vi "multi-function-fpga2.vi"() -> ()   [LabVIEW 2016]
uses:
  <vilib>/rvi/Emulation/niFpgaGetClockAttributes.vi
  <vilib>/rvi/Emulation/niFpgaSctlEmulationGetInTimedLoop.vi
  <vilib>/rvi/Emulation/niFpgaEmulationReportErrorSimple.vi
  <vilib>/rvi/eio/common/nirviEmuTemplateMethod_errors.vi
  <vilib>/rvi/Emulation/niFpgaCriticalErrorInLSC.vi
  <vilib>/eio/EIONode/EIONode.xnode
panel:
  out "input array":bool[](array[boolean])
  in  "Channel15":T1={"Ctrl"=enum."OFF", "high voltage"=3.5, "main input"=FALSE, "sub input"=FALSE, "low voltage"=0.0, "begin voltage"=0.0, "end voltage"=0.0, "step voltage"=0.0, "Set"=FALSE} {"step voltage" format="%#_17g"; "end voltage" format="%#_17g"; "begin voltage" format="%#_17g"; "low voltage" format="%#_17g"; "high voltage" format="%#_17g"}
  in  "Channel14":T1={"Ctrl"=enum."OFF", "high voltage"=3.5, "main input"=FALSE, "sub input"=FALSE, "low voltage"=0.0, "begin voltage"=0.0, "end voltage"=0.0, "step voltage"=0.0, "Set"=FALSE} {"step voltage" format="%#_17g"; "end voltage" format="%#_17g"; "begin voltage" format="%#_17g"; "low voltage" format="%#_17g"; "high voltage" format="%#_17g"}
  in  "Channel13":T1={"Ctrl"=enum."OFF", "high voltage"=3.5, "main input"=FALSE, "sub input"=FALSE, "low voltage"=0.0, "begin voltage"=0.0, "end voltage"=0.0, "step voltage"=0.0, "Set"=FALSE} {"step voltage" format="%#_17g"; "end voltage" format="%#_17g"; "begin voltage" format="%#_17g"; "low voltage" format="%#_17g"; "high voltage" format="%#_17g"}
  in  "Channel12":T1={"Ctrl"=enum."OFF", "high voltage"=3.5, "main input"=FALSE, "sub input"=FALSE, "low voltage"=0.0, "begin voltage"=0.0, "end voltage"=0.0, "step voltage"=0.0, "Set"=FALSE} {"step voltage" format="%#_17g"; "end voltage" format="%#_17g"; "begin voltage" format="%#_17g"; "low voltage" format="%#_17g"; "high voltage" format="%#_17g"}
  in  "Channel11":T1={"Ctrl"=enum."OFF", "high voltage"=3.5, "main input"=FALSE, "sub input"=FALSE, "low voltage"=0.0, "begin voltage"=0.0, "end voltage"=0.0, "step voltage"=0.0, "Set"=FALSE} {"step voltage" format="%#_17g"; "end voltage" format="%#_17g"; "begin voltage" format="%#_17g"; "low voltage" format="%#_17g"; "high voltage" format="%#_17g"}
  in  "Channel10":T1={"Ctrl"=enum."OFF", "high voltage"=3.5, "main input"=FALSE, "sub input"=FALSE, "low voltage"=0.0, "begin voltage"=0.0, "end voltage"=0.0, "step voltage"=0.0, "Set"=FALSE} {"step voltage" format="%#_17g"; "end voltage" format="%#_17g"; "begin voltage" format="%#_17g"; "low voltage" format="%#_17g"; "high voltage" format="%#_17g"}
  in  "Channel9":T1={"Ctrl"=enum."OFF", "high voltage"=3.5, "main input"=FALSE, "sub input"=FALSE, "low voltage"=0.0, "begin voltage"=0.0, "end voltage"=0.0, "step voltage"=0.0, "Set"=FALSE} {"step voltage" format="%#_17g"; "end voltage" format="%#_17g"; "begin voltage" format="%#_17g"; "low voltage" format="%#_17g"; "high voltage" format="%#_17g"}
  in  "Channel8":T1={"Ctrl"=enum."OFF", "high voltage"=3.5, "main input"=FALSE, "sub input"=FALSE, "low voltage"=0.0, "begin voltage"=0.0, "end voltage"=0.0, "step voltage"=0.0, "Set"=FALSE} {"step voltage" format="%#_17g"; "end voltage" format="%#_17g"; "begin voltage" format="%#_17g"; "low voltage" format="%#_17g"; "high voltage" format="%#_17g"}
  in  "Channel7":T1={"Ctrl"=enum."OFF", "high voltage"=3.5, "main input"=FALSE, "sub input"=FALSE, "low voltage"=0.0, "begin voltage"=0.0, "end voltage"=0.0, "step voltage"=0.0, "Set"=FALSE} {"step voltage" format="%#_17g"; "end voltage" format="%#_17g"; "begin voltage" format="%#_17g"; "low voltage" format="%#_17g"; "high voltage" format="%#_17g"}
  in  "Channel6":T1={"Ctrl"=enum."OFF", "high voltage"=3.5, "main input"=FALSE, "sub input"=FALSE, "low voltage"=0.0, "begin voltage"=0.0, "end voltage"=0.0, "step voltage"=0.0, "Set"=FALSE} {"step voltage" format="%#_17g"; "end voltage" format="%#_17g"; "begin voltage" format="%#_17g"; "low voltage" format="%#_17g"; "high voltage" format="%#_17g"}
  in  "Channel5":T1={"Ctrl"=enum."OFF", "high voltage"=3.5, "main input"=FALSE, "sub input"=FALSE, "low voltage"=0.0, "begin voltage"=0.0, "end voltage"=0.0, "step voltage"=0.0, "Set"=FALSE} {"step voltage" format="%#_17g"; "end voltage" format="%#_17g"; "begin voltage" format="%#_17g"; "low voltage" format="%#_17g"; "high voltage" format="%#_17g"}
  in  "Channel4":T1={"Ctrl"=enum."OFF", "high voltage"=3.5, "main input"=FALSE, "sub input"=FALSE, "low voltage"=0.0, "begin voltage"=0.0, "end voltage"=0.0, "step voltage"=0.0, "Set"=FALSE} {"step voltage" format="%#_17g"; "end voltage" format="%#_17g"; "begin voltage" format="%#_17g"; "low voltage" format="%#_17g"; "high voltage" format="%#_17g"}
  in  "Channel3":T1={"Ctrl"=enum."OFF", "high voltage"=3.5, "main input"=FALSE, "sub input"=FALSE, "low voltage"=0.0, "begin voltage"=0.0, "end voltage"=0.0, "step voltage"=0.0, "Set"=FALSE} {"step voltage" format="%#_17g"; "end voltage" format="%#_17g"; "begin voltage" format="%#_17g"; "low voltage" format="%#_17g"; "high voltage" format="%#_17g"}
  in  "Channel2":T1={"Ctrl"=enum."OFF", "high voltage"=3.5, "main input"=FALSE, "sub input"=FALSE, "low voltage"=0.0, "begin voltage"=0.0, "end voltage"=0.0, "step voltage"=0.0, "Set"=FALSE} {"step voltage" format="%#_17g"; "end voltage" format="%#_17g"; "begin voltage" format="%#_17g"; "low voltage" format="%#_17g"; "high voltage" format="%#_17g"}
  in  "Channel1":T1={"Ctrl"=enum."OFF", "high voltage"=3.5, "main input"=FALSE, "sub input"=FALSE, "low voltage"=0.0, "begin voltage"=0.0, "end voltage"=0.0, "step voltage"=0.0, "Set"=FALSE} {"step voltage" format="%#_17g"; "end voltage" format="%#_17g"; "begin voltage" format="%#_17g"; "low voltage" format="%#_17g"; "high voltage" format="%#_17g"}
  in  "Channel0":T1={"Ctrl"=enum."OFF", "high voltage"=3.5, "main input"=FALSE, "sub input"=FALSE, "low voltage"=0.0, "begin voltage"=0.0, "end voltage"=0.0, "step voltage"=0.0, "Set"=FALSE} {"step voltage" format="%#_17g"; "end voltage" format="%#_17g"; "begin voltage" format="%#_17g"; "low voltage" format="%#_17g"; "high voltage" format="%#_17g"}
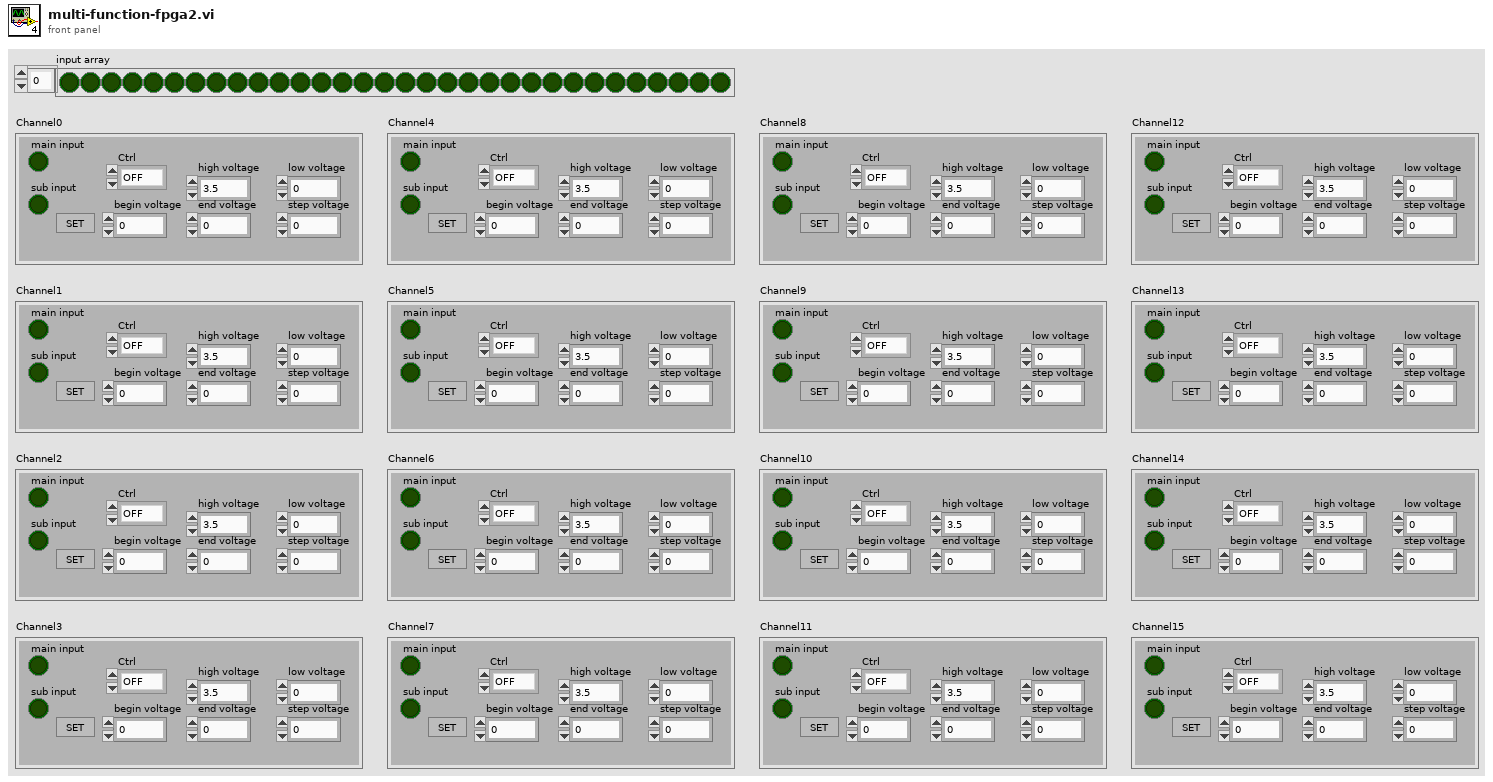
[diagram p1: front panel]
types:
  T1 = cluster{"Ctrl":enum16{"OFF", "SWITCH", "AND GATE", "OR GATE", "ITERATION"}, "high voltage":sgl, "main input":bool, "sub input":bool, "low voltage":sgl, "begin voltage":sgl, "end voltage":sgl, "step voltage":sgl, "Set":bool}
  T2 = enum16{"OFF", "SWITCH", "AND GATE", "OR GATE", "ITERATION"}
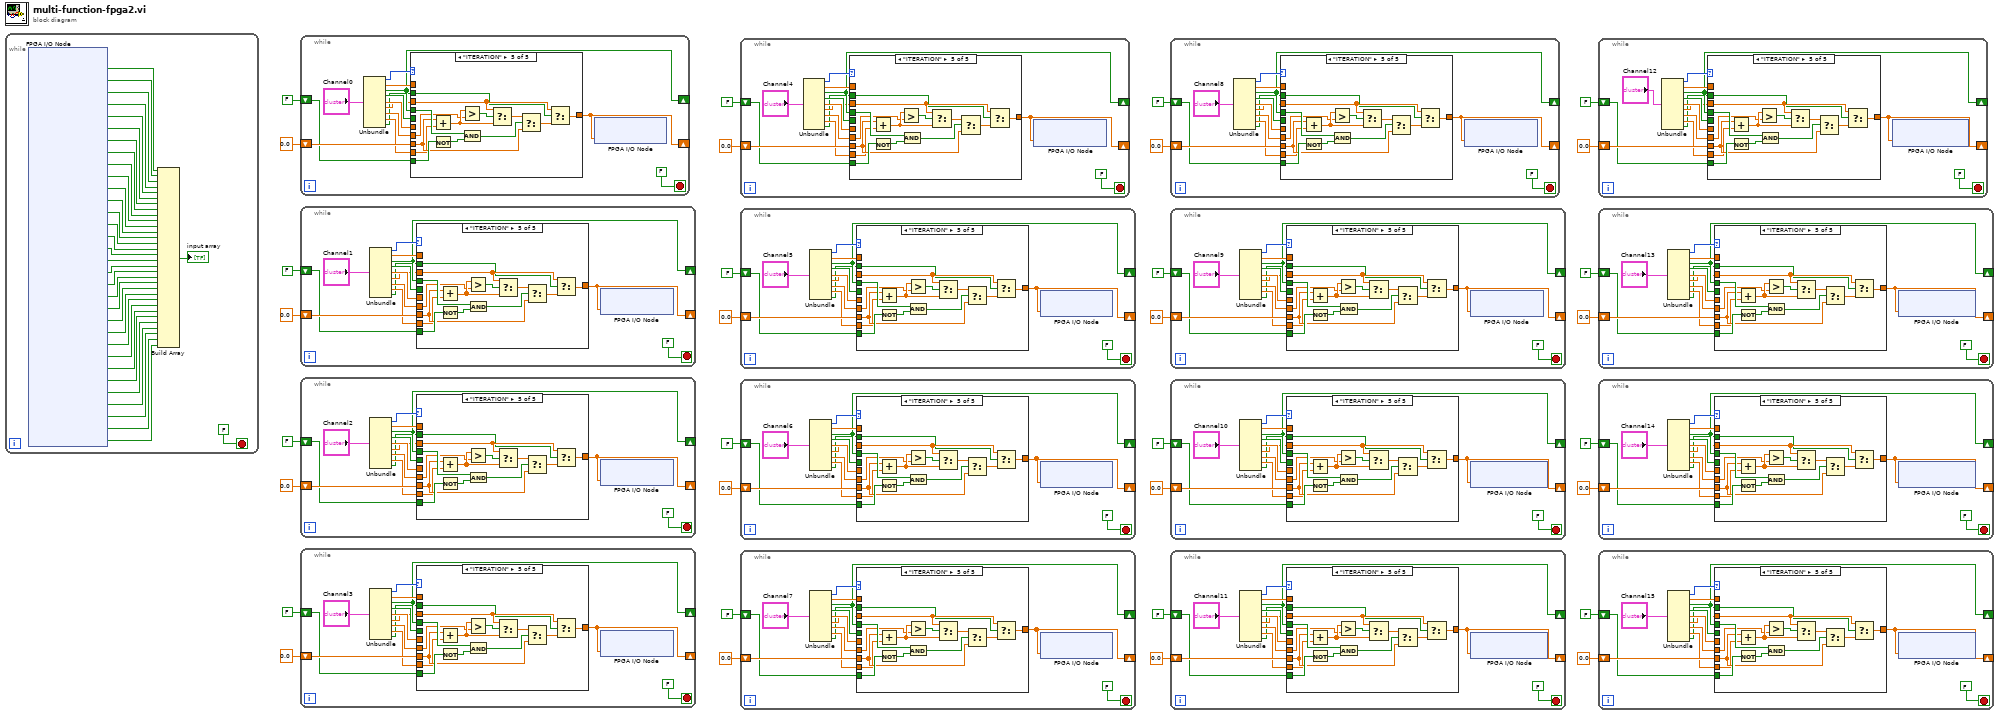
[diagram p0: block diagram]
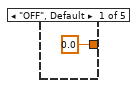
[diagram p2: hidden frame]
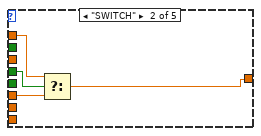
[diagram p3: hidden frame]
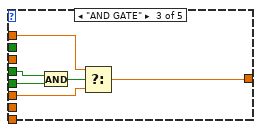
[diagram p4: hidden frame]
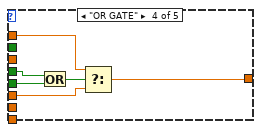
[diagram p5: hidden frame]
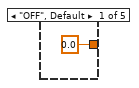
[diagram p6: hidden frame]
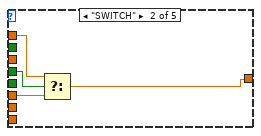
[diagram p7: hidden frame]
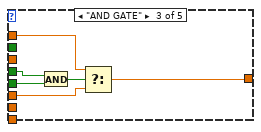
[diagram p8: hidden frame]
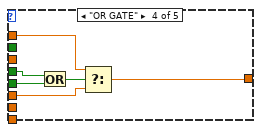
[diagram p9: hidden frame]
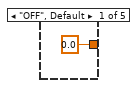
[diagram p10: hidden frame]
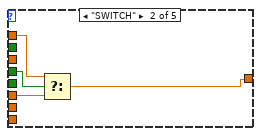
[diagram p11: hidden frame]
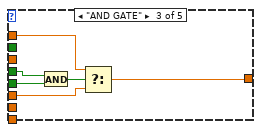
[diagram p12: hidden frame]
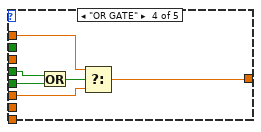
[diagram p13: hidden frame]
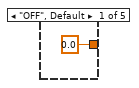
[diagram p14: hidden frame]
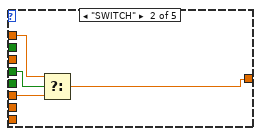
[diagram p15: hidden frame]
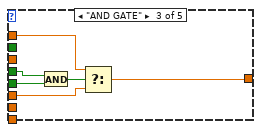
[diagram p16: hidden frame]
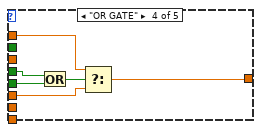
[diagram p17: hidden frame]
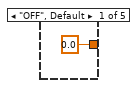
[diagram p18: hidden frame]
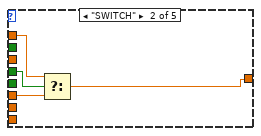
[diagram p19: hidden frame]
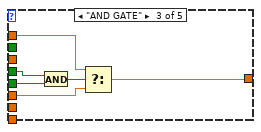
[diagram p20: hidden frame]
diagram:
  n1 = while {
    stop <- FALSE stop-if-true
    n2 = xnode "FPGA I/O Node"() -> ("Mod2/DIO0"=w65:bool, "Mod2/DIO1"=w64:bool, "Mod2/DIO2"=w63:bool, "Mod2/DIO3"=w62:bool, "Mod2/DIO4"=w61:bool, "Mod2/DIO5"=w60:bool, "Mod2/DIO6"=w59:bool, "Mod2/DIO7"=w58:bool, "Mod2/DIO8"=w57:bool, "Mod2/DIO9"=w56:bool, "Mod2/DIO10"=w55:bool, "Mod2/DIO11"=w54:bool, "Mod2/DIO12"=w53:bool, "Mod2/DIO13"=w52:bool, "Mod2/DIO14"=w51:bool, "Mod2/DIO15"=w50:bool, "Mod2/DIO16"=w49:bool, "Mod2/DIO17"=w48:bool, "Mod2/DIO18"=w47:bool, "Mod2/DIO19"=w46:bool, "Mod2/DIO20"=w45:bool, "Mod2/DIO21"=w44:bool, "Mod2/DIO22"=w43:bool, "Mod2/DIO23"=w42:bool, "Mod2/DIO24"=w41:bool, "Mod2/DIO25"=w40:bool, "Mod2/DIO26"=w39:bool, "Mod2/DIO27"=w38:bool, "Mod2/DIO28"=w37:bool, "Mod2/DIO29"=w36:bool, "Mod2/DIO30"=w35:bool, "Mod2/DIO31"=w34:bool)  [unwired: 32 in, 32 out]
    n3 = Build Array(w65, w64, w63, w62, w61, w60, w59, w58, w57, w56, w55, w54, w53, w52, w51, w50, w49, w48, w47, w46, w45, w44, w43, w42, w41, w40, w39, w38, w37, w36, w35, w34) -> (→"input array":bool[])
  }
  n4 = while {
    shift-right: [w78] -> _
    shift-left: sgl 0.0 -> [w79]
    shift-right: [w72] -> _
    shift-left: FALSE -> [w77]
    stop <- FALSE stop-if-true
    n5 = Unbundle("Channel0") -> ("Ctrl"=w75:T2, "high voltage"=w74:sgl, "main input"=w72:bool, "sub input"=w71:bool, "low voltage"=w73:sgl, "begin voltage"=w68:sgl, "end voltage"=w69:sgl, "step voltage"=w70:sgl, "Set"=w67:bool)
    n6 = case shown="\"ITERATION\"" w75 {
      tunnel: w71 -> [_ _ w90 w96 _]
      tunnel: w72 -> [_ w84 w91 w97 w110]
      tunnel: [sgl 0.0 ("Mod4/AO0") w85 w88 w94 w102] -> w78
      tunnel: w74 -> [_ w83 w87 w93 _]
      tunnel: w73 -> [_ w82 w86 w92 _]
      tunnel: w79 -> [_ _ _ _ w104]
      tunnel: w77 -> [_ _ _ _ w111]
      tunnel: w70 -> [_ _ _ _ w101]
      tunnel: w69 -> [_ _ _ _ w100]
      tunnel: w68 -> [_ _ _ _ w99]
      tunnel: w67 -> [_ _ _ _ w98]
      frame "OFF", Default {
      }
      frame "SWITCH" {
        n7 = Select(t=w83, s=w84, f=w82) -> (s? t:f=w85:sgl)
      }
      frame "AND GATE" {
        n8 = And(x=w91, y=w90) -> (x .and. y?=w89:bool)
        n9 = Select(t=w87, s=w89, f=w86) -> (s? t:f=w88:sgl)
      }
      frame "OR GATE" {
        n10 = Or(x=w97, y=w96) -> (x .or. y?=w95:bool)
        n11 = Select(t=w93, s=w95, f=w92) -> (s? t:f=w94:sgl)
      }
      frame "ITERATION" {
        n12 = Add(x=w104, y=w101) -> (x+y=w106:sgl)
        n13 = Not(x=w111) -> (.not. x?=w109:bool)
        n14 = Greater?(x=w106, y=w100) -> (0:w107:bool)
        n15 = And(x=w110, y=w109) -> (x .and. y?=w108:bool)
        n16 = Select(t=w99, s=w107, f=w106) -> (s? t:f=w105:sgl)
        n17 = Select(t=w105, s=w108, f=w104) -> (s? t:f=w103:sgl)
        n18 = Select(t=w99, s=w98, f=w103) -> (s? t:f=w102:sgl)
      }
    }
    n19 = xnode "FPGA I/O Node"("Mod4/AO0"=w78) -> ()  [unwired: 1 in, 1 out]
  }
  n20 = while {
    shift-right: [w123] -> _
    shift-left: sgl 0.0 -> [w124]
    shift-right: [w117] -> _
    shift-left: FALSE -> [w122]
    stop <- FALSE stop-if-true
    n21 = Unbundle("Channel1") -> ("Ctrl"=w120:T2, "high voltage"=w119:sgl, "main input"=w117:bool, "sub input"=w116:bool, "low voltage"=w118:sgl, "begin voltage"=w113:sgl, "end voltage"=w114:sgl, "step voltage"=w115:sgl, "Set"=w112:bool)
    n22 = case shown="\"ITERATION\"" w120 {
      tunnel: w116 -> [_ _ w135 w141 _]
      tunnel: w117 -> [_ w129 w136 w142 w155]
      tunnel: [sgl 0.0 ("Mod4/AO0") w130 w133 w139 w147] -> w123
      tunnel: w119 -> [_ w128 w132 w138 _]
      tunnel: w118 -> [_ w127 w131 w137 _]
      tunnel: w124 -> [_ _ _ _ w149]
      tunnel: w122 -> [_ _ _ _ w156]
      tunnel: w115 -> [_ _ _ _ w146]
      tunnel: w114 -> [_ _ _ _ w145]
      tunnel: w113 -> [_ _ _ _ w144]
      tunnel: w112 -> [_ _ _ _ w143]
      frame "OFF", Default {
      }
      frame "SWITCH" {
        n23 = Select(t=w128, s=w129, f=w127) -> (s? t:f=w130:sgl)
      }
      frame "AND GATE" {
        n24 = And(x=w136, y=w135) -> (x .and. y?=w134:bool)
        n25 = Select(t=w132, s=w134, f=w131) -> (s? t:f=w133:sgl)
      }
      frame "OR GATE" {
        n26 = Or(x=w142, y=w141) -> (x .or. y?=w140:bool)
        n27 = Select(t=w138, s=w140, f=w137) -> (s? t:f=w139:sgl)
      }
      frame "ITERATION" {
        n28 = Add(x=w149, y=w146) -> (x+y=w151:sgl)
        n29 = Not(x=w156) -> (.not. x?=w154:bool)
        n30 = Greater?(x=w151, y=w145) -> (0:w152:bool)
        n31 = And(x=w155, y=w154) -> (x .and. y?=w153:bool)
        n32 = Select(t=w144, s=w152, f=w151) -> (s? t:f=w150:sgl)
        n33 = Select(t=w150, s=w153, f=w149) -> (s? t:f=w148:sgl)
        n34 = Select(t=w144, s=w143, f=w148) -> (s? t:f=w147:sgl)
      }
    }
    n35 = xnode "FPGA I/O Node"("Mod4/AO1"=w123) -> ()  [unwired: 1 in, 1 out]
  }
  n36 = while {
    shift-right: [w168] -> _
    shift-left: sgl 0.0 -> [w169]
    shift-right: [w162] -> _
    shift-left: FALSE -> [w167]
    stop <- FALSE stop-if-true
    n37 = Unbundle("Channel2") -> ("Ctrl"=w165:T2, "high voltage"=w164:sgl, "main input"=w162:bool, "sub input"=w161:bool, "low voltage"=w163:sgl, "begin voltage"=w158:sgl, "end voltage"=w159:sgl, "step voltage"=w160:sgl, "Set"=w157:bool)
    n38 = case shown="\"ITERATION\"" w165 {
      tunnel: w161 -> [_ _ w180 w186 _]
      tunnel: w162 -> [_ w174 w181 w187 w200]
      tunnel: [sgl 0.0 ("Mod4/AO0") w175 w178 w184 w192] -> w168
      tunnel: w164 -> [_ w173 w177 w183 _]
      tunnel: w163 -> [_ w172 w176 w182 _]
      tunnel: w169 -> [_ _ _ _ w194]
      tunnel: w167 -> [_ _ _ _ w201]
      tunnel: w160 -> [_ _ _ _ w191]
      tunnel: w159 -> [_ _ _ _ w190]
      tunnel: w158 -> [_ _ _ _ w189]
      tunnel: w157 -> [_ _ _ _ w188]
      frame "OFF", Default {
      }
      frame "SWITCH" {
        n39 = Select(t=w173, s=w174, f=w172) -> (s? t:f=w175:sgl)
      }
      frame "AND GATE" {
        n40 = And(x=w181, y=w180) -> (x .and. y?=w179:bool)
        n41 = Select(t=w177, s=w179, f=w176) -> (s? t:f=w178:sgl)
      }
      frame "OR GATE" {
        n42 = Or(x=w187, y=w186) -> (x .or. y?=w185:bool)
        n43 = Select(t=w183, s=w185, f=w182) -> (s? t:f=w184:sgl)
      }
      frame "ITERATION" {
        n44 = Add(x=w194, y=w191) -> (x+y=w196:sgl)
        n45 = Not(x=w201) -> (.not. x?=w199:bool)
        n46 = Greater?(x=w196, y=w190) -> (0:w197:bool)
        n47 = And(x=w200, y=w199) -> (x .and. y?=w198:bool)
        n48 = Select(t=w189, s=w197, f=w196) -> (s? t:f=w195:sgl)
        n49 = Select(t=w195, s=w198, f=w194) -> (s? t:f=w193:sgl)
        n50 = Select(t=w189, s=w188, f=w193) -> (s? t:f=w192:sgl)
      }
    }
    n51 = xnode "FPGA I/O Node"("Mod4/AO2"=w168) -> ()  [unwired: 1 in, 1 out]
  }
  n52 = while {
    shift-right: [w213] -> _
    shift-left: sgl 0.0 -> [w214]
    shift-right: [w207] -> _
    shift-left: FALSE -> [w212]
    stop <- FALSE stop-if-true
    n53 = Unbundle("Channel3") -> ("Ctrl"=w210:T2, "high voltage"=w209:sgl, "main input"=w207:bool, "sub input"=w206:bool, "low voltage"=w208:sgl, "begin voltage"=w203:sgl, "end voltage"=w204:sgl, "step voltage"=w205:sgl, "Set"=w202:bool)
    n54 = case shown="\"ITERATION\"" w210 {
      tunnel: w206 -> [_ _ w225 w231 _]
      tunnel: w207 -> [_ w219 w226 w232 w245]
      tunnel: [sgl 0.0 ("Mod4/AO0") w220 w223 w229 w237] -> w213
      tunnel: w209 -> [_ w218 w222 w228 _]
      tunnel: w208 -> [_ w217 w221 w227 _]
      tunnel: w214 -> [_ _ _ _ w239]
      tunnel: w212 -> [_ _ _ _ w246]
      tunnel: w205 -> [_ _ _ _ w236]
      tunnel: w204 -> [_ _ _ _ w235]
      tunnel: w203 -> [_ _ _ _ w234]
      tunnel: w202 -> [_ _ _ _ w233]
      frame "OFF", Default {
      }
      frame "SWITCH" {
        n55 = Select(t=w218, s=w219, f=w217) -> (s? t:f=w220:sgl)
      }
      frame "AND GATE" {
        n56 = And(x=w226, y=w225) -> (x .and. y?=w224:bool)
        n57 = Select(t=w222, s=w224, f=w221) -> (s? t:f=w223:sgl)
      }
      frame "OR GATE" {
        n58 = Or(x=w232, y=w231) -> (x .or. y?=w230:bool)
        n59 = Select(t=w228, s=w230, f=w227) -> (s? t:f=w229:sgl)
      }
      frame "ITERATION" {
        n60 = Add(x=w239, y=w236) -> (x+y=w241:sgl)
        n61 = Not(x=w246) -> (.not. x?=w244:bool)
        n62 = Greater?(x=w241, y=w235) -> (0:w242:bool)
        n63 = And(x=w245, y=w244) -> (x .and. y?=w243:bool)
        n64 = Select(t=w234, s=w242, f=w241) -> (s? t:f=w240:sgl)
        n65 = Select(t=w240, s=w243, f=w239) -> (s? t:f=w238:sgl)
        n66 = Select(t=w234, s=w233, f=w238) -> (s? t:f=w237:sgl)
      }
    }
    n67 = xnode "FPGA I/O Node"("Mod4/AO3"=w213) -> ()  [unwired: 1 in, 1 out]
  }
  n68 = while {
    shift-right: [w258] -> _
    shift-left: sgl 0.0 -> [w259]
    shift-right: [w252] -> _
    shift-left: FALSE -> [w257]
    stop <- FALSE stop-if-true
    n69 = Unbundle("Channel4") -> ("Ctrl"=w255:T2, "high voltage"=w254:sgl, "main input"=w252:bool, "sub input"=w251:bool, "low voltage"=w253:sgl, "begin voltage"=w248:sgl, "end voltage"=w249:sgl, "step voltage"=w250:sgl, "Set"=w247:bool)
    n70 = case shown="\"ITERATION\"" w255 {
      tunnel: w251 -> [_ _ w270 w276 _]
      tunnel: w252 -> [_ w264 w271 w277 w290]
      tunnel: [sgl 0.0 ("Mod4/AO0") w265 w268 w274 w282] -> w258
      tunnel: w254 -> [_ w263 w267 w273 _]
      tunnel: w253 -> [_ w262 w266 w272 _]
      tunnel: w259 -> [_ _ _ _ w284]
      tunnel: w257 -> [_ _ _ _ w291]
      tunnel: w250 -> [_ _ _ _ w281]
      tunnel: w249 -> [_ _ _ _ w280]
      tunnel: w248 -> [_ _ _ _ w279]
      tunnel: w247 -> [_ _ _ _ w278]
      frame "OFF", Default {
      }
      frame "SWITCH" {
        n71 = Select(t=w263, s=w264, f=w262) -> (s? t:f=w265:sgl)
      }
      frame "AND GATE" {
        n72 = And(x=w271, y=w270) -> (x .and. y?=w269:bool)
        n73 = Select(t=w267, s=w269, f=w266) -> (s? t:f=w268:sgl)
      }
      frame "OR GATE" {
        n74 = Or(x=w277, y=w276) -> (x .or. y?=w275:bool)
        n75 = Select(t=w273, s=w275, f=w272) -> (s? t:f=w274:sgl)
      }
      frame "ITERATION" {
        n76 = Add(x=w284, y=w281) -> (x+y=w286:sgl)
        n77 = Not(x=w291) -> (.not. x?=w289:bool)
        n78 = Greater?(x=w286, y=w280) -> (0:w287:bool)
        n79 = And(x=w290, y=w289) -> (x .and. y?=w288:bool)
        n80 = Select(t=w279, s=w287, f=w286) -> (s? t:f=w285:sgl)
        n81 = Select(t=w285, s=w288, f=w284) -> (s? t:f=w283:sgl)
        n82 = Select(t=w279, s=w278, f=w283) -> (s? t:f=w282:sgl)
      }
    }
    n83 = xnode "FPGA I/O Node"("Mod4/AO4"=w258) -> ()  [unwired: 1 in, 1 out]
  }
  n84 = while {
    shift-right: [w303] -> _
    shift-left: sgl 0.0 -> [w304]
    shift-right: [w297] -> _
    shift-left: FALSE -> [w302]
    stop <- FALSE stop-if-true
    n85 = Unbundle("Channel5") -> ("Ctrl"=w300:T2, "high voltage"=w299:sgl, "main input"=w297:bool, "sub input"=w296:bool, "low voltage"=w298:sgl, "begin voltage"=w293:sgl, "end voltage"=w294:sgl, "step voltage"=w295:sgl, "Set"=w292:bool)
    n86 = case shown="\"ITERATION\"" w300 {
      tunnel: w296 -> [_ _ w315 w321 _]
      tunnel: w297 -> [_ w309 w316 w322 w335]
      tunnel: [sgl 0.0 ("Mod4/AO0") w310 w313 w319 w327] -> w303
      tunnel: w299 -> [_ w308 w312 w318 _]
      tunnel: w298 -> [_ w307 w311 w317 _]
      tunnel: w304 -> [_ _ _ _ w329]
      tunnel: w302 -> [_ _ _ _ w336]
      tunnel: w295 -> [_ _ _ _ w326]
      tunnel: w294 -> [_ _ _ _ w325]
      tunnel: w293 -> [_ _ _ _ w324]
      tunnel: w292 -> [_ _ _ _ w323]
      frame "OFF", Default {
      }
      frame "SWITCH" {
        n87 = Select(t=w308, s=w309, f=w307) -> (s? t:f=w310:sgl)
      }
      frame "AND GATE" {
        n88 = And(x=w316, y=w315) -> (x .and. y?=w314:bool)
        n89 = Select(t=w312, s=w314, f=w311) -> (s? t:f=w313:sgl)
      }
      frame "OR GATE" {
        n90 = Or(x=w322, y=w321) -> (x .or. y?=w320:bool)
        n91 = Select(t=w318, s=w320, f=w317) -> (s? t:f=w319:sgl)
      }
      frame "ITERATION" {
        n92 = Add(x=w329, y=w326) -> (x+y=w331:sgl)
        n93 = Not(x=w336) -> (.not. x?=w334:bool)
        n94 = Greater?(x=w331, y=w325) -> (0:w332:bool)
        n95 = And(x=w335, y=w334) -> (x .and. y?=w333:bool)
        n96 = Select(t=w324, s=w332, f=w331) -> (s? t:f=w330:sgl)
        n97 = Select(t=w330, s=w333, f=w329) -> (s? t:f=w328:sgl)
        n98 = Select(t=w324, s=w323, f=w328) -> (s? t:f=w327:sgl)
      }
    }
    n99 = xnode "FPGA I/O Node"("Mod4/AO5"=w303) -> ()  [unwired: 1 in, 1 out]
  }
  n100 = while {
    shift-right: [w348] -> _
    shift-left: sgl 0.0 -> [w349]
    shift-right: [w342] -> _
    shift-left: FALSE -> [w347]
    stop <- FALSE stop-if-true
    n101 = Unbundle("Channel6") -> ("Ctrl"=w345:T2, "high voltage"=w344:sgl, "main input"=w342:bool, "sub input"=w341:bool, "low voltage"=w343:sgl, "begin voltage"=w338:sgl, "end voltage"=w339:sgl, "step voltage"=w340:sgl, "Set"=w337:bool)
    n102 = case shown="\"ITERATION\"" w345 {
      tunnel: w341 -> [_ _ w360 w366 _]
      tunnel: w342 -> [_ w354 w361 w367 w380]
      tunnel: [sgl 0.0 ("Mod4/AO0") w355 w358 w364 w372] -> w348
      tunnel: w344 -> [_ w353 w357 w363 _]
      tunnel: w343 -> [_ w352 w356 w362 _]
      tunnel: w349 -> [_ _ _ _ w374]
      tunnel: w347 -> [_ _ _ _ w381]
      tunnel: w340 -> [_ _ _ _ w371]
      tunnel: w339 -> [_ _ _ _ w370]
      tunnel: w338 -> [_ _ _ _ w369]
      tunnel: w337 -> [_ _ _ _ w368]
      frame "OFF", Default {
      }
      frame "SWITCH" {
        n103 = Select(t=w353, s=w354, f=w352) -> (s? t:f=w355:sgl)
      }
      frame "AND GATE" {
        n104 = And(x=w361, y=w360) -> (x .and. y?=w359:bool)
        n105 = Select(t=w357, s=w359, f=w356) -> (s? t:f=w358:sgl)
      }
      frame "OR GATE" {
        n106 = Or(x=w367, y=w366) -> (x .or. y?=w365:bool)
        n107 = Select(t=w363, s=w365, f=w362) -> (s? t:f=w364:sgl)
      }
      frame "ITERATION" {
        n108 = Add(x=w374, y=w371) -> (x+y=w376:sgl)
        n109 = Not(x=w381) -> (.not. x?=w379:bool)
        n110 = Greater?(x=w376, y=w370) -> (0:w377:bool)
        n111 = And(x=w380, y=w379) -> (x .and. y?=w378:bool)
        n112 = Select(t=w369, s=w377, f=w376) -> (s? t:f=w375:sgl)
        n113 = Select(t=w375, s=w378, f=w374) -> (s? t:f=w373:sgl)
        n114 = Select(t=w369, s=w368, f=w373) -> (s? t:f=w372:sgl)
      }
    }
    n115 = xnode "FPGA I/O Node"("Mod4/AO6"=w348) -> ()  [unwired: 1 in, 1 out]
  }
  n116 = while {
    shift-right: [w393] -> _
    shift-left: sgl 0.0 -> [w394]
    shift-right: [w387] -> _
    shift-left: FALSE -> [w392]
    stop <- FALSE stop-if-true
    n117 = Unbundle("Channel7") -> ("Ctrl"=w390:T2, "high voltage"=w389:sgl, "main input"=w387:bool, "sub input"=w386:bool, "low voltage"=w388:sgl, "begin voltage"=w383:sgl, "end voltage"=w384:sgl, "step voltage"=w385:sgl, "Set"=w382:bool)
    n118 = case shown="\"ITERATION\"" w390 {
      tunnel: w386 -> [_ _ w405 w411 _]
      tunnel: w387 -> [_ w399 w406 w412 w425]
      tunnel: [sgl 0.0 ("Mod4/AO0") w400 w403 w409 w417] -> w393
      tunnel: w389 -> [_ w398 w402 w408 _]
      tunnel: w388 -> [_ w397 w401 w407 _]
      tunnel: w394 -> [_ _ _ _ w419]
      tunnel: w392 -> [_ _ _ _ w426]
      tunnel: w385 -> [_ _ _ _ w416]
      tunnel: w384 -> [_ _ _ _ w415]
      tunnel: w383 -> [_ _ _ _ w414]
      tunnel: w382 -> [_ _ _ _ w413]
      frame "OFF", Default {
      }
      frame "SWITCH" {
        n119 = Select(t=w398, s=w399, f=w397) -> (s? t:f=w400:sgl)
      }
      frame "AND GATE" {
        n120 = And(x=w406, y=w405) -> (x .and. y?=w404:bool)
        n121 = Select(t=w402, s=w404, f=w401) -> (s? t:f=w403:sgl)
      }
      frame "OR GATE" {
        n122 = Or(x=w412, y=w411) -> (x .or. y?=w410:bool)
        n123 = Select(t=w408, s=w410, f=w407) -> (s? t:f=w409:sgl)
      }
      frame "ITERATION" {
        n124 = Add(x=w419, y=w416) -> (x+y=w421:sgl)
        n125 = Not(x=w426) -> (.not. x?=w424:bool)
        n126 = Greater?(x=w421, y=w415) -> (0:w422:bool)
        n127 = And(x=w425, y=w424) -> (x .and. y?=w423:bool)
        n128 = Select(t=w414, s=w422, f=w421) -> (s? t:f=w420:sgl)
        n129 = Select(t=w420, s=w423, f=w419) -> (s? t:f=w418:sgl)
        n130 = Select(t=w414, s=w413, f=w418) -> (s? t:f=w417:sgl)
      }
    }
    n131 = xnode "FPGA I/O Node"("Mod4/AO7"=w393) -> ()  [unwired: 1 in, 1 out]
  }
  n132 = while {
    shift-right: [w438] -> _
    shift-left: sgl 0.0 -> [w439]
    shift-right: [w432] -> _
    shift-left: FALSE -> [w437]
    stop <- FALSE stop-if-true
    n133 = Unbundle("Channel8") -> ("Ctrl"=w435:T2, "high voltage"=w434:sgl, "main input"=w432:bool, "sub input"=w431:bool, "low voltage"=w433:sgl, "begin voltage"=w428:sgl, "end voltage"=w429:sgl, "step voltage"=w430:sgl, "Set"=w427:bool)
    n134 = case shown="\"ITERATION\"" w435 {
      tunnel: w431 -> [_ _ w450 w456 _]
      tunnel: w432 -> [_ w444 w451 w457 w470]
      tunnel: [sgl 0.0 ("Mod4/AO0") w445 w448 w454 w462] -> w438
      tunnel: w434 -> [_ w443 w447 w453 _]
      tunnel: w433 -> [_ w442 w446 w452 _]
      tunnel: w439 -> [_ _ _ _ w464]
      tunnel: w437 -> [_ _ _ _ w471]
      tunnel: w430 -> [_ _ _ _ w461]
      tunnel: w429 -> [_ _ _ _ w460]
      tunnel: w428 -> [_ _ _ _ w459]
      tunnel: w427 -> [_ _ _ _ w458]
      frame "OFF", Default {
      }
      frame "SWITCH" {
        n135 = Select(t=w443, s=w444, f=w442) -> (s? t:f=w445:sgl)
      }
      frame "AND GATE" {
        n136 = And(x=w451, y=w450) -> (x .and. y?=w449:bool)
        n137 = Select(t=w447, s=w449, f=w446) -> (s? t:f=w448:sgl)
      }
      frame "OR GATE" {
        n138 = Or(x=w457, y=w456) -> (x .or. y?=w455:bool)
        n139 = Select(t=w453, s=w455, f=w452) -> (s? t:f=w454:sgl)
      }
      frame "ITERATION" {
        n140 = Add(x=w464, y=w461) -> (x+y=w466:sgl)
        n141 = Not(x=w471) -> (.not. x?=w469:bool)
        n142 = Greater?(x=w466, y=w460) -> (0:w467:bool)
        n143 = And(x=w470, y=w469) -> (x .and. y?=w468:bool)
        n144 = Select(t=w459, s=w467, f=w466) -> (s? t:f=w465:sgl)
        n145 = Select(t=w465, s=w468, f=w464) -> (s? t:f=w463:sgl)
        n146 = Select(t=w459, s=w458, f=w463) -> (s? t:f=w462:sgl)
      }
    }
    n147 = xnode "FPGA I/O Node"("Mod4/AO8"=w438) -> ()  [unwired: 1 in, 1 out]
  }
  n148 = while {
    shift-right: [w483] -> _
    shift-left: sgl 0.0 -> [w484]
    shift-right: [w477] -> _
    shift-left: FALSE -> [w482]
    stop <- FALSE stop-if-true
    n149 = Unbundle("Channel9") -> ("Ctrl"=w480:T2, "high voltage"=w479:sgl, "main input"=w477:bool, "sub input"=w476:bool, "low voltage"=w478:sgl, "begin voltage"=w473:sgl, "end voltage"=w474:sgl, "step voltage"=w475:sgl, "Set"=w472:bool)
    n150 = case shown="\"ITERATION\"" w480 {
      tunnel: w476 -> [_ _ w495 w501 _]
      tunnel: w477 -> [_ w489 w496 w502 w515]
      tunnel: [sgl 0.0 ("Mod4/AO0") w490 w493 w499 w507] -> w483
      tunnel: w479 -> [_ w488 w492 w498 _]
      tunnel: w478 -> [_ w487 w491 w497 _]
      tunnel: w484 -> [_ _ _ _ w509]
      tunnel: w482 -> [_ _ _ _ w516]
      tunnel: w475 -> [_ _ _ _ w506]
      tunnel: w474 -> [_ _ _ _ w505]
      tunnel: w473 -> [_ _ _ _ w504]
      tunnel: w472 -> [_ _ _ _ w503]
      frame "OFF", Default {
      }
      frame "SWITCH" {
        n151 = Select(t=w488, s=w489, f=w487) -> (s? t:f=w490:sgl)
      }
      frame "AND GATE" {
        n152 = And(x=w496, y=w495) -> (x .and. y?=w494:bool)
        n153 = Select(t=w492, s=w494, f=w491) -> (s? t:f=w493:sgl)
      }
      frame "OR GATE" {
        n154 = Or(x=w502, y=w501) -> (x .or. y?=w500:bool)
        n155 = Select(t=w498, s=w500, f=w497) -> (s? t:f=w499:sgl)
      }
      frame "ITERATION" {
        n156 = Add(x=w509, y=w506) -> (x+y=w511:sgl)
        n157 = Not(x=w516) -> (.not. x?=w514:bool)
        n158 = Greater?(x=w511, y=w505) -> (0:w512:bool)
        n159 = And(x=w515, y=w514) -> (x .and. y?=w513:bool)
        n160 = Select(t=w504, s=w512, f=w511) -> (s? t:f=w510:sgl)
        n161 = Select(t=w510, s=w513, f=w509) -> (s? t:f=w508:sgl)
        n162 = Select(t=w504, s=w503, f=w508) -> (s? t:f=w507:sgl)
      }
    }
    n163 = xnode "FPGA I/O Node"("Mod4/AO9"=w483) -> ()  [unwired: 1 in, 1 out]
  }
  n164 = while {
    shift-right: [w528] -> _
    shift-left: sgl 0.0 -> [w529]
    shift-right: [w522] -> _
    shift-left: FALSE -> [w527]
    stop <- FALSE stop-if-true
    n165 = Unbundle("Channel10") -> ("Ctrl"=w525:T2, "high voltage"=w524:sgl, "main input"=w522:bool, "sub input"=w521:bool, "low voltage"=w523:sgl, "begin voltage"=w518:sgl, "end voltage"=w519:sgl, "step voltage"=w520:sgl, "Set"=w517:bool)
    n166 = case shown="\"ITERATION\"" w525 {
      tunnel: w521 -> [_ _ w540 w546 _]
      tunnel: w522 -> [_ w534 w541 w547 w560]
      tunnel: [sgl 0.0 ("Mod4/AO0") w535 w538 w544 w552] -> w528
      tunnel: w524 -> [_ w533 w537 w543 _]
      tunnel: w523 -> [_ w532 w536 w542 _]
      tunnel: w529 -> [_ _ _ _ w554]
      tunnel: w527 -> [_ _ _ _ w561]
      tunnel: w520 -> [_ _ _ _ w551]
      tunnel: w519 -> [_ _ _ _ w550]
      tunnel: w518 -> [_ _ _ _ w549]
      tunnel: w517 -> [_ _ _ _ w548]
      frame "OFF", Default {
      }
      frame "SWITCH" {
        n167 = Select(t=w533, s=w534, f=w532) -> (s? t:f=w535:sgl)
      }
      frame "AND GATE" {
        n168 = And(x=w541, y=w540) -> (x .and. y?=w539:bool)
        n169 = Select(t=w537, s=w539, f=w536) -> (s? t:f=w538:sgl)
      }
      frame "OR GATE" {
        n170 = Or(x=w547, y=w546) -> (x .or. y?=w545:bool)
        n171 = Select(t=w543, s=w545, f=w542) -> (s? t:f=w544:sgl)
      }
      frame "ITERATION" {
        n172 = Add(x=w554, y=w551) -> (x+y=w556:sgl)
        n173 = Not(x=w561) -> (.not. x?=w559:bool)
        n174 = Greater?(x=w556, y=w550) -> (0:w557:bool)
        n175 = And(x=w560, y=w559) -> (x .and. y?=w558:bool)
        n176 = Select(t=w549, s=w557, f=w556) -> (s? t:f=w555:sgl)
        n177 = Select(t=w555, s=w558, f=w554) -> (s? t:f=w553:sgl)
        n178 = Select(t=w549, s=w548, f=w553) -> (s? t:f=w552:sgl)
      }
    }
    n179 = xnode "FPGA I/O Node"("Mod4/AO10"=w528) -> ()  [unwired: 1 in, 1 out]
  }
  n180 = while {
    shift-right: [w573] -> _
    shift-left: sgl 0.0 -> [w574]
    shift-right: [w567] -> _
    shift-left: FALSE -> [w572]
    stop <- FALSE stop-if-true
    n181 = Unbundle("Channel11") -> ("Ctrl"=w570:T2, "high voltage"=w569:sgl, "main input"=w567:bool, "sub input"=w566:bool, "low voltage"=w568:sgl, "begin voltage"=w563:sgl, "end voltage"=w564:sgl, "step voltage"=w565:sgl, "Set"=w562:bool)
    n182 = case shown="\"ITERATION\"" w570 {
      tunnel: w566 -> [_ _ w585 w591 _]
      tunnel: w567 -> [_ w579 w586 w592 w605]
      tunnel: [sgl 0.0 ("Mod4/AO0") w580 w583 w589 w597] -> w573
      tunnel: w569 -> [_ w578 w582 w588 _]
      tunnel: w568 -> [_ w577 w581 w587 _]
      tunnel: w574 -> [_ _ _ _ w599]
      tunnel: w572 -> [_ _ _ _ w606]
      tunnel: w565 -> [_ _ _ _ w596]
      tunnel: w564 -> [_ _ _ _ w595]
      tunnel: w563 -> [_ _ _ _ w594]
      tunnel: w562 -> [_ _ _ _ w593]
      frame "OFF", Default {
      }
      frame "SWITCH" {
        n183 = Select(t=w578, s=w579, f=w577) -> (s? t:f=w580:sgl)
      }
      frame "AND GATE" {
        n184 = And(x=w586, y=w585) -> (x .and. y?=w584:bool)
        n185 = Select(t=w582, s=w584, f=w581) -> (s? t:f=w583:sgl)
      }
      frame "OR GATE" {
        n186 = Or(x=w592, y=w591) -> (x .or. y?=w590:bool)
        n187 = Select(t=w588, s=w590, f=w587) -> (s? t:f=w589:sgl)
      }
      frame "ITERATION" {
        n188 = Add(x=w599, y=w596) -> (x+y=w601:sgl)
        n189 = Not(x=w606) -> (.not. x?=w604:bool)
        n190 = Greater?(x=w601, y=w595) -> (0:w602:bool)
        n191 = And(x=w605, y=w604) -> (x .and. y?=w603:bool)
        n192 = Select(t=w594, s=w602, f=w601) -> (s? t:f=w600:sgl)
        n193 = Select(t=w600, s=w603, f=w599) -> (s? t:f=w598:sgl)
        n194 = Select(t=w594, s=w593, f=w598) -> (s? t:f=w597:sgl)
      }
    }
    n195 = xnode "FPGA I/O Node"("Mod4/AO11"=w573) -> ()  [unwired: 1 in, 1 out]
  }
  n196 = while {
    shift-right: [w618] -> _
    shift-left: sgl 0.0 -> [w619]
    shift-right: [w612] -> _
    shift-left: FALSE -> [w617]
    stop <- FALSE stop-if-true
    n197 = Unbundle("Channel12") -> ("Ctrl"=w615:T2, "high voltage"=w614:sgl, "main input"=w612:bool, "sub input"=w611:bool, "low voltage"=w613:sgl, "begin voltage"=w608:sgl, "end voltage"=w609:sgl, "step voltage"=w610:sgl, "Set"=w607:bool)
    n198 = case shown="\"ITERATION\"" w615 {
      tunnel: w611 -> [_ _ w630 w636 _]
      tunnel: w612 -> [_ w624 w631 w637 w650]
      tunnel: [sgl 0.0 ("Mod4/AO0") w625 w628 w634 w642] -> w618
      tunnel: w614 -> [_ w623 w627 w633 _]
      tunnel: w613 -> [_ w622 w626 w632 _]
      tunnel: w619 -> [_ _ _ _ w644]
      tunnel: w617 -> [_ _ _ _ w651]
      tunnel: w610 -> [_ _ _ _ w641]
      tunnel: w609 -> [_ _ _ _ w640]
      tunnel: w608 -> [_ _ _ _ w639]
      tunnel: w607 -> [_ _ _ _ w638]
      frame "OFF", Default {
      }
      frame "SWITCH" {
        n199 = Select(t=w623, s=w624, f=w622) -> (s? t:f=w625:sgl)
      }
      frame "AND GATE" {
        n200 = And(x=w631, y=w630) -> (x .and. y?=w629:bool)
        n201 = Select(t=w627, s=w629, f=w626) -> (s? t:f=w628:sgl)
      }
      frame "OR GATE" {
        n202 = Or(x=w637, y=w636) -> (x .or. y?=w635:bool)
        n203 = Select(t=w633, s=w635, f=w632) -> (s? t:f=w634:sgl)
      }
      frame "ITERATION" {
        n204 = Add(x=w644, y=w641) -> (x+y=w646:sgl)
        n205 = Not(x=w651) -> (.not. x?=w649:bool)
        n206 = Greater?(x=w646, y=w640) -> (0:w647:bool)
        n207 = And(x=w650, y=w649) -> (x .and. y?=w648:bool)
        n208 = Select(t=w639, s=w647, f=w646) -> (s? t:f=w645:sgl)
        n209 = Select(t=w645, s=w648, f=w644) -> (s? t:f=w643:sgl)
        n210 = Select(t=w639, s=w638, f=w643) -> (s? t:f=w642:sgl)
      }
    }
    n211 = xnode "FPGA I/O Node"("Mod4/AO12"=w618) -> ()  [unwired: 1 in, 1 out]
  }
  n212 = while {
    shift-right: [w663] -> _
    shift-left: sgl 0.0 -> [w664]
    shift-right: [w657] -> _
    shift-left: FALSE -> [w662]
    stop <- FALSE stop-if-true
    n213 = Unbundle("Channel13") -> ("Ctrl"=w660:T2, "high voltage"=w659:sgl, "main input"=w657:bool, "sub input"=w656:bool, "low voltage"=w658:sgl, "begin voltage"=w653:sgl, "end voltage"=w654:sgl, "step voltage"=w655:sgl, "Set"=w652:bool)
    n214 = case shown="\"ITERATION\"" w660 {
      tunnel: w656 -> [_ _ w675 w681 _]
      tunnel: w657 -> [_ w669 w676 w682 w695]
      tunnel: [sgl 0.0 ("Mod4/AO0") w670 w673 w679 w687] -> w663
      tunnel: w659 -> [_ w668 w672 w678 _]
      tunnel: w658 -> [_ w667 w671 w677 _]
      tunnel: w664 -> [_ _ _ _ w689]
      tunnel: w662 -> [_ _ _ _ w696]
      tunnel: w655 -> [_ _ _ _ w686]
      tunnel: w654 -> [_ _ _ _ w685]
      tunnel: w653 -> [_ _ _ _ w684]
      tunnel: w652 -> [_ _ _ _ w683]
      frame "OFF", Default {
      }
      frame "SWITCH" {
        n215 = Select(t=w668, s=w669, f=w667) -> (s? t:f=w670:sgl)
      }
      frame "AND GATE" {
        n216 = And(x=w676, y=w675) -> (x .and. y?=w674:bool)
        n217 = Select(t=w672, s=w674, f=w671) -> (s? t:f=w673:sgl)
      }
      frame "OR GATE" {
        n218 = Or(x=w682, y=w681) -> (x .or. y?=w680:bool)
        n219 = Select(t=w678, s=w680, f=w677) -> (s? t:f=w679:sgl)
      }
      frame "ITERATION" {
        n220 = Add(x=w689, y=w686) -> (x+y=w691:sgl)
        n221 = Not(x=w696) -> (.not. x?=w694:bool)
        n222 = Greater?(x=w691, y=w685) -> (0:w692:bool)
        n223 = And(x=w695, y=w694) -> (x .and. y?=w693:bool)
        n224 = Select(t=w684, s=w692, f=w691) -> (s? t:f=w690:sgl)
        n225 = Select(t=w690, s=w693, f=w689) -> (s? t:f=w688:sgl)
        n226 = Select(t=w684, s=w683, f=w688) -> (s? t:f=w687:sgl)
      }
    }
    n227 = xnode "FPGA I/O Node"("Mod4/AO13"=w663) -> ()  [unwired: 1 in, 1 out]
  }
  n228 = while {
    shift-right: [w708] -> _
    shift-left: sgl 0.0 -> [w709]
    shift-right: [w702] -> _
    shift-left: FALSE -> [w707]
    stop <- FALSE stop-if-true
    n229 = Unbundle("Channel14") -> ("Ctrl"=w705:T2, "high voltage"=w704:sgl, "main input"=w702:bool, "sub input"=w701:bool, "low voltage"=w703:sgl, "begin voltage"=w698:sgl, "end voltage"=w699:sgl, "step voltage"=w700:sgl, "Set"=w697:bool)
    n230 = case shown="\"ITERATION\"" w705 {
      tunnel: w701 -> [_ _ w720 w726 _]
      tunnel: w702 -> [_ w714 w721 w727 w740]
      tunnel: [sgl 0.0 ("Mod4/AO0") w715 w718 w724 w732] -> w708
      tunnel: w704 -> [_ w713 w717 w723 _]
      tunnel: w703 -> [_ w712 w716 w722 _]
      tunnel: w709 -> [_ _ _ _ w734]
      tunnel: w707 -> [_ _ _ _ w741]
      tunnel: w700 -> [_ _ _ _ w731]
      tunnel: w699 -> [_ _ _ _ w730]
      tunnel: w698 -> [_ _ _ _ w729]
      tunnel: w697 -> [_ _ _ _ w728]
      frame "OFF", Default {
      }
      frame "SWITCH" {
        n231 = Select(t=w713, s=w714, f=w712) -> (s? t:f=w715:sgl)
      }
      frame "AND GATE" {
        n232 = And(x=w721, y=w720) -> (x .and. y?=w719:bool)
        n233 = Select(t=w717, s=w719, f=w716) -> (s? t:f=w718:sgl)
      }
      frame "OR GATE" {
        n234 = Or(x=w727, y=w726) -> (x .or. y?=w725:bool)
        n235 = Select(t=w723, s=w725, f=w722) -> (s? t:f=w724:sgl)
      }
      frame "ITERATION" {
        n236 = Add(x=w734, y=w731) -> (x+y=w736:sgl)
        n237 = Not(x=w741) -> (.not. x?=w739:bool)
        n238 = Greater?(x=w736, y=w730) -> (0:w737:bool)
        n239 = And(x=w740, y=w739) -> (x .and. y?=w738:bool)
        n240 = Select(t=w729, s=w737, f=w736) -> (s? t:f=w735:sgl)
        n241 = Select(t=w735, s=w738, f=w734) -> (s? t:f=w733:sgl)
        n242 = Select(t=w729, s=w728, f=w733) -> (s? t:f=w732:sgl)
      }
    }
    n243 = xnode "FPGA I/O Node"("Mod4/AO14"=w708) -> ()  [unwired: 1 in, 1 out]
  }
  n244 = while {
    shift-right: [w753] -> _
    shift-left: sgl 0.0 -> [w754]
    shift-right: [w747] -> _
    shift-left: FALSE -> [w752]
    stop <- FALSE stop-if-true
    n245 = Unbundle("Channel15") -> ("Ctrl"=w750:T2, "high voltage"=w749:sgl, "main input"=w747:bool, "sub input"=w746:bool, "low voltage"=w748:sgl, "begin voltage"=w743:sgl, "end voltage"=w744:sgl, "step voltage"=w745:sgl, "Set"=w742:bool)
    n246 = case shown="\"ITERATION\"" w750 {
      tunnel: w746 -> [_ _ w765 w771 _]
      tunnel: w747 -> [_ w759 w766 w772 w785]
      tunnel: [sgl 0.0 ("Mod4/AO0") w760 w763 w769 w777] -> w753
      tunnel: w749 -> [_ w758 w762 w768 _]
      tunnel: w748 -> [_ w757 w761 w767 _]
      tunnel: w754 -> [_ _ _ _ w779]
      tunnel: w752 -> [_ _ _ _ w786]
      tunnel: w745 -> [_ _ _ _ w776]
      tunnel: w744 -> [_ _ _ _ w775]
      tunnel: w743 -> [_ _ _ _ w774]
      tunnel: w742 -> [_ _ _ _ w773]
      frame "OFF", Default {
      }
      frame "SWITCH" {
        n247 = Select(t=w758, s=w759, f=w757) -> (s? t:f=w760:sgl)
      }
      frame "AND GATE" {
        n248 = And(x=w766, y=w765) -> (x .and. y?=w764:bool)
        n249 = Select(t=w762, s=w764, f=w761) -> (s? t:f=w763:sgl)
      }
      frame "OR GATE" {
        n250 = Or(x=w772, y=w771) -> (x .or. y?=w770:bool)
        n251 = Select(t=w768, s=w770, f=w767) -> (s? t:f=w769:sgl)
      }
      frame "ITERATION" {
        n252 = Add(x=w779, y=w776) -> (x+y=w781:sgl)
        n253 = Not(x=w786) -> (.not. x?=w784:bool)
        n254 = Greater?(x=w781, y=w775) -> (0:w782:bool)
        n255 = And(x=w785, y=w784) -> (x .and. y?=w783:bool)
        n256 = Select(t=w774, s=w782, f=w781) -> (s? t:f=w780:sgl)
        n257 = Select(t=w780, s=w783, f=w779) -> (s? t:f=w778:sgl)
        n258 = Select(t=w774, s=w773, f=w778) -> (s? t:f=w777:sgl)
      }
    }
    n259 = xnode "FPGA I/O Node"("Mod4/AO15"=w753) -> ()  [unwired: 1 in, 1 out]
  }
